vi "Newmark-Exceptions.vi"(0 "Exception IN":bool[](array[boolean])=[FALSE, FALSE, FALSE, FALSE], 2 "New Exception":i32=-1, 13 "Make False":bool[](array[boolean])=[FALSE, FALSE, FALSE, FALSE]) -> (4 "Exception OUT":bool[](array[boolean]), 6 "Command Error":bool=TRUE, 8 "Slip/Stall":bool=TRUE, 10 "Overtravel":bool=TRUE, 15 "Done":bool=TRUE)   [LabVIEW 2011]
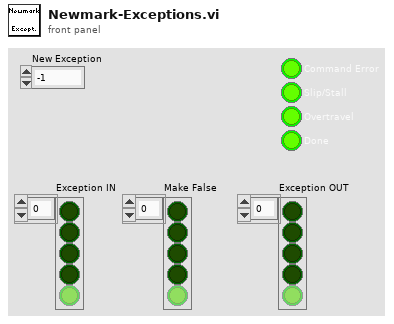
[diagram p1: front panel]
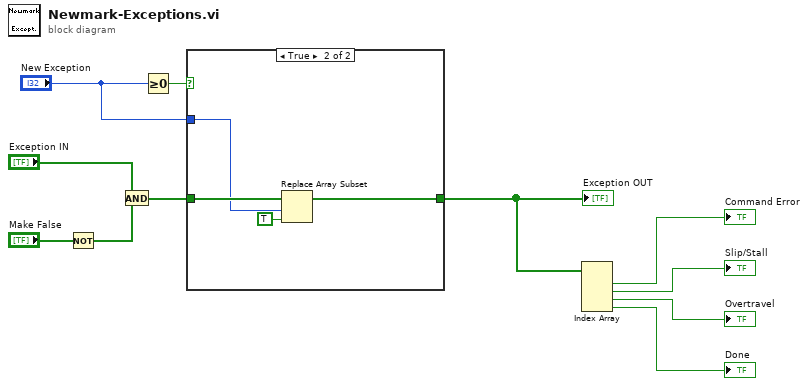
[diagram p0: block diagram]
diagram:
  n1 = Not(x="Make False") -> (.not. x?=w9:bool[])
  n2 = And(x="Exception IN", y=w9) -> (x .and. y?=w7:bool[])
  n3 = Greater Or Equal To 0?(x="New Exception") -> (x >= 0?=w8:bool)
  n4 = case shown="True" w8 {
    tunnel: [w12 w15] -> w1
    tunnel: w7 -> [w12 w16]
    tunnel: "New Exception" -> [_ w13]
    frame False {
    }
    frame True {
      n5 = Replace Array Subset(array=w16, new element=TRUE ("new element/subarray"), index=w13) -> (w15:bool[])
    }
  }
  "Exception OUT" <- w1
  n6 = Index Array(array=w1) -> (element #1=→"Command Error":bool, element #2=→"Slip/Stall":bool, element #3=→"Overtravel":bool, element #4=→"Done":bool)  [unwired: 4 in]
